vi "SVT Gain and Phase.vi"   [LabVIEW 2017, in "SoundVib_SingleTone.lvlib"]
doc: "Computes the gain and phase between <B>stimulus signal X</B> and <B>response signal Y</B> at the fundamental frequency. This VI returns the detected fundamental frequency, detected response amplitude, gain, and phase lag. This VI does not maintain state internally; you can use this VI in a loop to process multiple blocks. Wire data to the <B>stimulus signal X [Eux]</B> and <B>response signal Y [Euy]</B> inputs to determine the polymorphic instance to use or manually select the instance."
uses:
  <vilib>/addons/Sound and Vibration/svt_Single Tone Measurements/SoundVib_SingleTone.lvlib
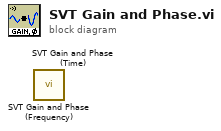
[diagram p0: block diagram]
diagram:
  n1 = call <vilib>:"SVT Gain and Phase (Frequency).vi"() -> ()  [unwired: 12 in, 8 out]
  n2 = call <vilib>:"SVT Gain and Phase (Time).vi"() -> ()  [unwired: 12 in, 8 out]
